vi "Get_Data.vi"(0 "Divide in":refnum<class "Divide.lvclass">, 11 "Error In":errorcluster) -> (4 "Divide out":refnum<class "Divide.lvclass">, 15 "Error Out":errorcluster)   [LabVIEW 2020, in "Divide.lvclass"]
doc: "Method to get the object data from the UI method."
uses:
  Divide.lvclass
  D:/Github Projects/LV_Assignment/Tasks/A18/A18/Classes/Arithmetic_Operations/Arithmetic_Operations.lvclass
  Arithmetic_Operations/Arithmetic_Operations.lvclass
  Divide.lvclass/Divide.ctl
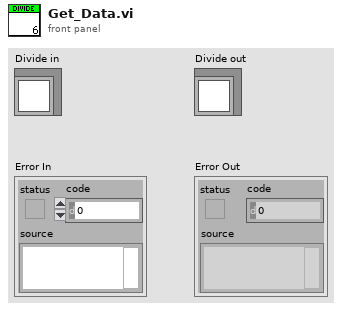
[diagram p1: front panel]
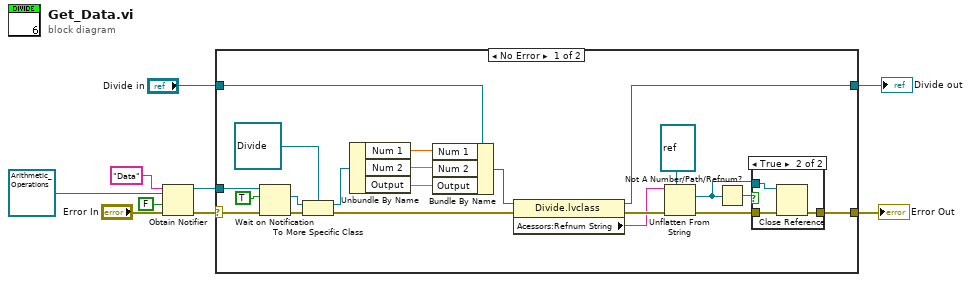
[diagram p0: block diagram]
diagram:
  n1 = Obtain Notifier(name (unnamed)="Data", notification data type=refnum<class "Arithmetic_Operations.lvclass"> refnum ("Arithmetic_Operations.lvclass"), create if not found? (T)=FALSE, error in (no error)="Error In") -> (notifier out=w7:refnum<notifier>, error out=w5:errorcluster)  [unwired: 1 out]
  n2 = case shown="No Error" w5 {
    selector: w5 -> [w26 w36]
    tunnel: [w10 w36] -> w9
    tunnel: [w16 w35] -> w2
    tunnel: "Divide in" -> [w30 w35]
    tunnel: w7 -> [w24 _]
    frame No Error {
      n3 = Wait on Notification(notifier=w24, ignore previous (F)=TRUE, error in (no error)=w26) -> (notification=w22:refnum<class "Arithmetic_Operations.lvclass">, error out=w25:errorcluster)  [unwired: 1 in, 2 out]
      n4 = To More Specific Class(target class=refnum<class "Divide.lvclass"> refnum ("Divide.lvclass"), reference=w22, error in=w25) -> (specific class reference=w21:refnum<class "Divide.lvclass">, error out=w23:errorcluster)
      n5 = Unbundle By Name(w21) -> ("Num 1"=w29:dbl, "Num 2"=w28:dbl, "Output"=w27:dbl)
      n6 = Bundle By Name(cluster=w30, "Num 1"=w29, "Num 2"=w28, "Output"=w27) -> (w17:refnum<class "Divide.lvclass">)
      n7 = property class="Divide.lvclass"(reference=w17, error in=w23) -> (reference out=w16:refnum<class "Divide.lvclass">, error out=w18:errorcluster, "Acessors:Refnum String"=w14:string)
      n8 = Unflatten From String(type=refnum<vi> refnum ("reference out"), binary string=w14, error in (no error)=w18) -> (value=w11:refnum<vi>, error out=w12:errorcluster)  [unwired: 2 in, 1 out]
      n9 = Not A Number/Path/Refnum?(number/path/refnum=w11) -> (NaN/Path/Refnum?=w13:bool)
      n10 = case shown="True" w13 {
        tunnel: [w31 w34] -> w10
        tunnel: w12 -> [w31 w33]
        tunnel: w11 -> [_ w32]
        frame False {
        }
        frame True {
          n11 = Close Reference(reference=w32, error in (no error)=w33) -> (error out=w34:errorcluster)
        }
      }
    }
    frame Error {
    }
  }
  "Divide out" <- w2
  "Error Out" <- w9
